vi "nominal run search.vi"(0 "client":i32, 1 "search_text":string, 2 "label":string, 3 "property_key":string, 4 "property_value":string, 5 "run_number":u32, 6 "start_after_ms":dbl, 7 "error in (no error)":errorcluster, 8 "has_start_after":bool, 9 "end_before_ms":dbl, 10 "has_end_before":bool, 11 "out_list":i32, 12 "out_count":u32) -> (14 "out_count out":u32, 17 "out_list out":i32, 20 "function return":i32, 27 "error out":errorcluster)   [LabVIEW 2020, in "client.lvlib"]
doc: "int32_t nominal_run_search(int32_t client,\n const char *search_text,\n const char *label,\n const char *property_key,\n const char *property_value,\n uint32_t run_number,\n double start_after_ms,\n bool has_start_after,\n double end_before_ms,\n bool has_end_before,\n int32_t *out_list,\n uint32_t *out_count);"
uses:
  client.lvlib
  bin/nominalClient_64.dll
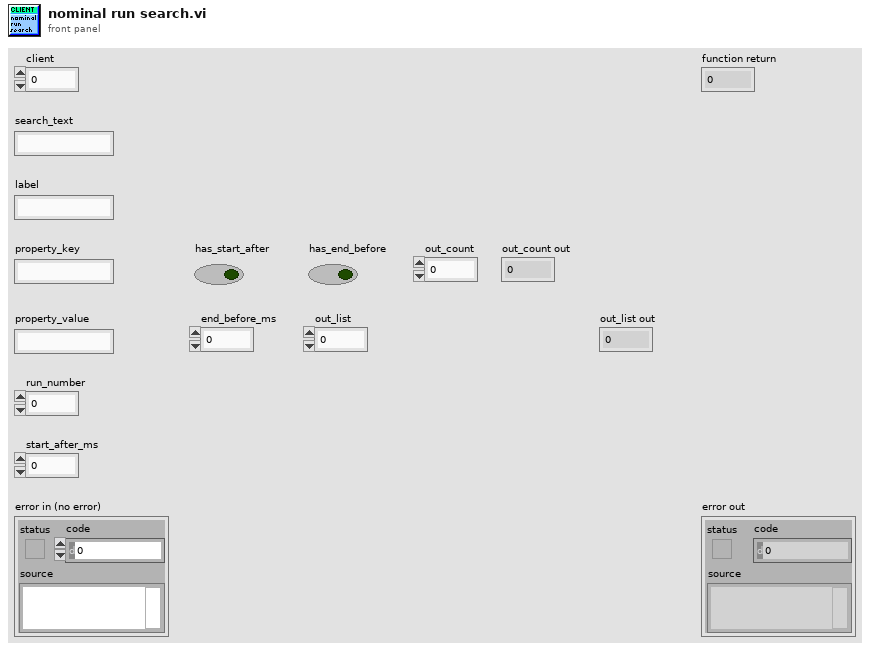
[diagram p1: front panel]
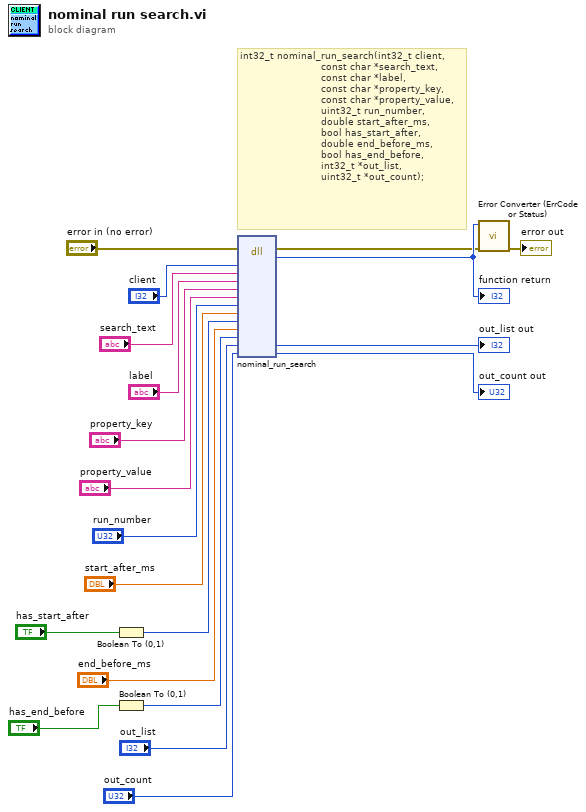
[diagram p0: block diagram]
diagram:
  # "int32_t nominal_run_search(int32_t client,\n                           const char *search_text,\n                           const char *label,\n                           const char *property_key,\n                           const char *property_value,\n                           uint32_t run_number,\n                           double start_after_ms,\n                           bool has_start_after,\n                           double end_before_ms,\n                           bool has_end_before,\n                           int32_t *out_list,\n                           uint32_t *out_count);"
  n1 = Boolean To (0,1)(Boolean="has_start_after") -> (0, 1=w11:i16)
  n2 = Boolean To (0,1)(Boolean="has_end_before") -> (0, 1=w8:i16)
  n3 = dll-call lib="C:/code/labview-client-rs/lv_src/bin/nominalClient_*.*" fn="nominal_run_search"(error in="error in (no error)", "client"="client", "search_text"="search_text", "label"="label", "property_key"="property_key", "property_value"="property_value", "run_number"="run_number", "start_after_ms"="start_after_ms", "has_start_after"=w11, "end_before_ms"="end_before_ms", "has_end_before"=w8, "out_list"="out_list", "out_count"="out_count") -> (error out=w2:errorcluster, w20:i32, "out_list"=→"out_list out":i32, "out_count"=→"out_count out":u32)  [unwired: 12 in, 1 out]
  "function return" <- w20
  n4 = call "Error Converter (ErrCode or Status).vi"("error in (no error)"=w2, "error code"=w20) -> ("error out"=→"error out":errorcluster)  [unwired: 9 in]
